vi "SVL Set dB Reference (1 Ch).vi"(8 "error in (no error)":errorcluster, 10 "dB reference [EU]":dbl=1.0 format="%^.1e", 11 "scaled signal in [EU]":waveform(dbl)={"t0"=timestamp(0 s since 1904-01-01), "dt"=0.0, "Y"=[]}) -> (0 "error out":errorcluster, 3 "scaled signal out [EU]":waveform(dbl))   [LabVIEW 2017]
doc: "Sets the specified <B>dB reference [EU]</B> as an attribute in the <B>scaled signal out [EU]</B> waveform. <B>dB reference [EU]</B> is used for all downstream conversions to dB. Wire data to the <B>scaled signal in [EU]</B> input to determine the polymorphic instance to use or manually select the instance."
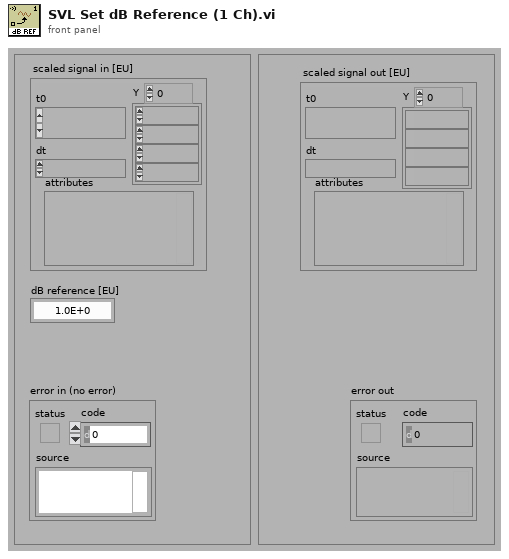
[diagram p1: front panel]
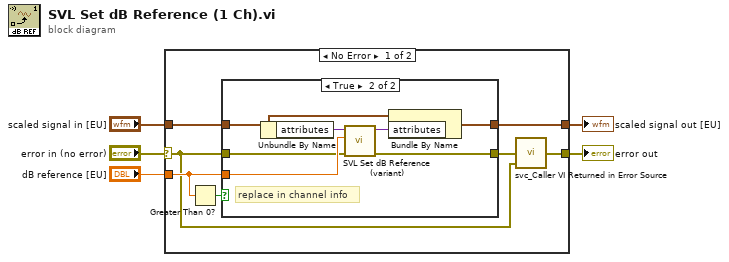
[diagram p0: block diagram]
diagram:
  n1 = case shown="No Error" "error in (no error)" {
    selector: "error in (no error)" -> [w6 w23]
    tunnel: "scaled signal in [EU]" -> [w12 w22]
    tunnel: [w8 w23] -> w4
    tunnel: [w9 w22] -> w3
    tunnel: "dB reference [EU]" -> [w11 _]
    frame No Error {
      n2 = Greater Than 0?(x=w11) -> (x > 0?=w10:bool)
      n3 = case shown="True" w10 {
        tunnel: w12 -> [w13 w18]
        tunnel: w6 -> [w14 w15]
        tunnel: [w14 w17] -> w7
        tunnel: [w13 w19] -> w9
        tunnel: w11 -> [_ w16]
        frame False {
        }
        frame True {
          # "replace in channel info"
          n4 = Unbundle By Name(w18) -> ("attributes"=w21:variant)
          n5 = call <vilib>:"SVL Set dB Reference (variant).vi"("error in (no error)"=w15, "dB reference [EU]"=w16, "attributes in"=w21) -> ("error out"=w17:errorcluster, "attributes out"=w20:variant)  [unwired: 7 in]
          n6 = Bundle By Name(cluster=w18, "attributes"=w20) -> (w19:waveform(dbl))
        }
      }
      n7 = call <vilib>:"svc_Caller VI Returned in Error Source.vi"("warning input to caller"=w6, "error in (no error)"=w7) -> ("error out"=w8:errorcluster)  [unwired: 3 in]
    }
    frame Error {
    }
  }
  "scaled signal out [EU]" <- w3
  "error out" <- w4
